vi "push.vi"(1 "ptr_write":i32, 2 "Data in":dbl[][](array[numeric])) -> (0 "Data":dbl[][](array[numeric]))   [LabVIEW 2013]
uses:
  GlobleVar/segment_size.vi
  GlobleVar/Data.vi
  GlobleVar/ptr_write.vi
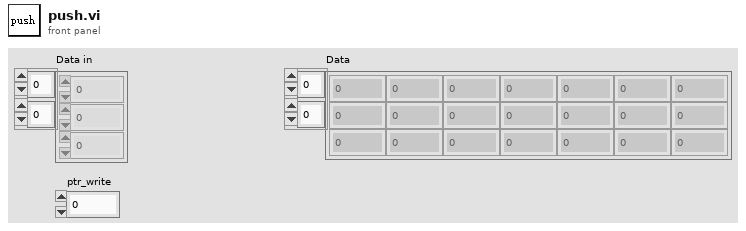
[diagram p1: front panel]
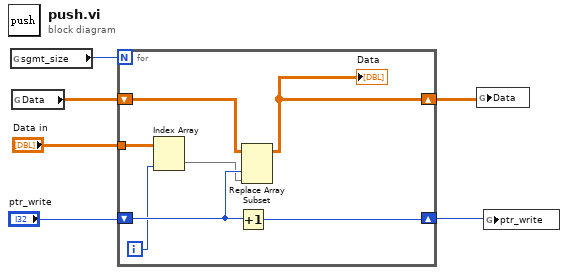
[diagram p0: block diagram]
diagram:
  n1 = global read "segment_size.vi" "sgmt_size"() -> (w6:i32)
  n2 = global read "Data.vi" "Data"() -> (w5:dbl[][])
  n3 = for {
    N: w6 -> [_]
    shift-right: [w13] -> w4
    shift-left: "ptr_write" -> [w12]
    tunnel: "Data in" -> [w10]
    shift-right: [w7] -> w2
    shift-left: w5 -> [w11]
    i -> [w8]
    n4 = Index Array(array=w10, index (col)=w8) -> (element=w9:dbl[])  [unwired: 1 in]
    n5 = Increment(x=w12) -> (x+1=w13:i32)
    n6 = Replace Array Subset(array=w11, new element=w9, index (col)=w12) -> (w7:dbl[][])  [unwired: 1 in]
    "Data" <- w7
  }
  n7 = global write "Data.vi" "Data"(w2) -> ()
  n8 = global write "ptr_write.vi" "ptr_write"(w4) -> ()
